vi "Keysight DAQ970-Example-Mantoles.vi"(5 "error in (no error)":errorcluster {"code" format="%.0x"}) -> (19 "error out":errorcluster)   [LabVIEW 2020, in "Keysight DAQ970.lvlib"]
doc: "Initializes the driver, reads a few Identity attributes, and checks the instrument error queue."
uses:
  Keysight DAQ970.lvlib
panel:
  out "Field Count":i32
  in  "MaxTimeMilliseconds":i32=5000
  in  "Sweep Count":i32=2 format="%.0g"
  in  "Resolution":dbl=0.01
  in  "Range":dbl=10.0
  out "muxSlot":i32=200
  out "dacSlot":i32=100
  out "Slot (Slot1)":i32
  out "Module ID":string
  out "ChannelList":string="(@305)"
  in  "Voltage":dbl=2.345
  out "Output":string
  out "Info":T1
  out "Simulate":bool
  in  "Simulate":bool=TRUE
  in  "Select ?":bool=TRUE
  in  "DAQ Resource":string="MyVisaAlias" caption="Instrument Resource"
  in  "Options String":string="DriverSetup= "
  # "Setup Scan"
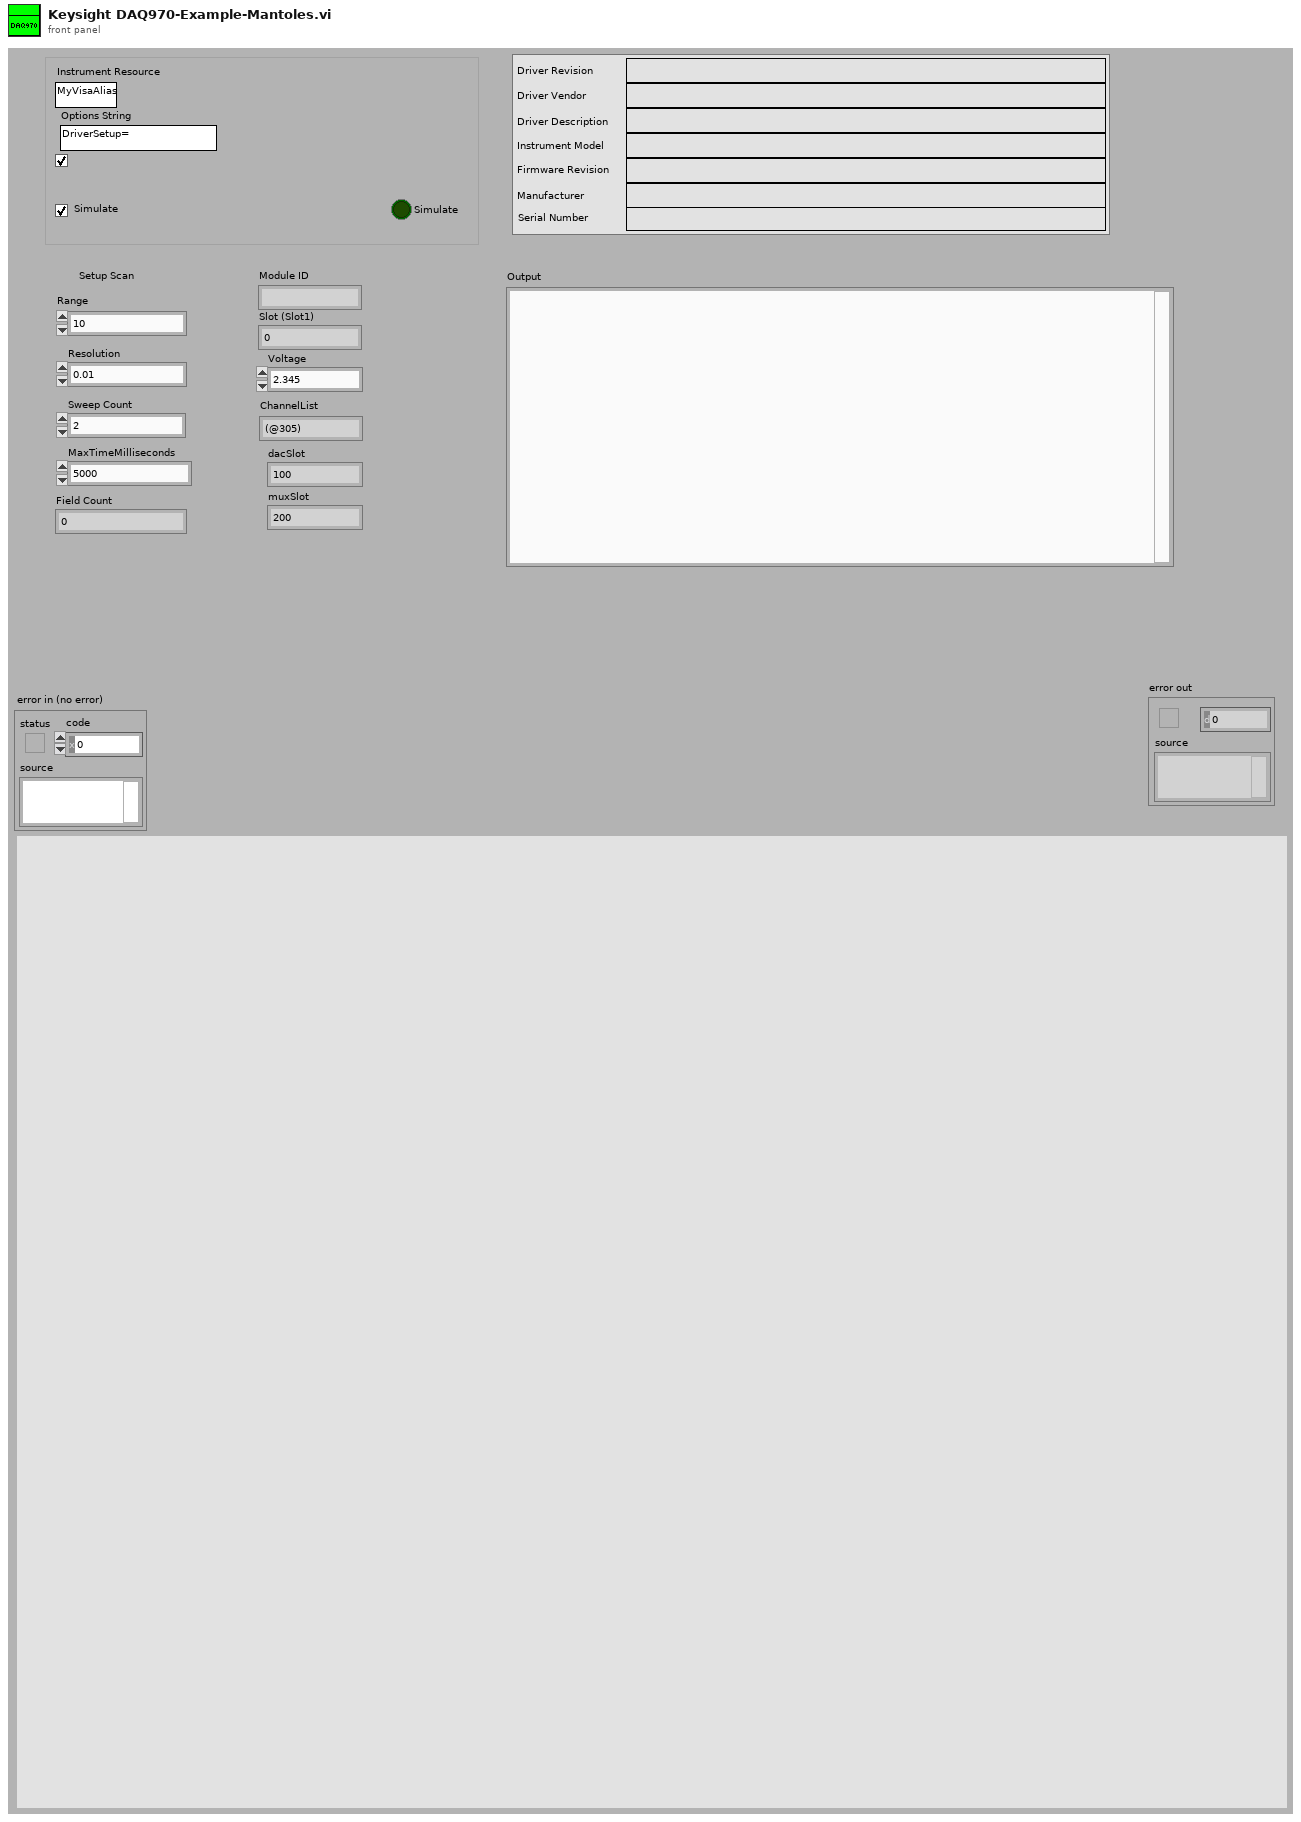
[diagram p1: front panel]
types:
  T1 = cluster{"Driver Revision":string, "Driver Vendor":string, "Driver Description":string, "Instrument Model":string, "Firmware Revision":string, "Instrument Model 2":string, "Firmware Revision 2":string}
  T2 = cluster{"[0]":string, "[1]":string, "[2]":string, "[3]":string, "[4]":string, "[5]":string, "[6]":string}
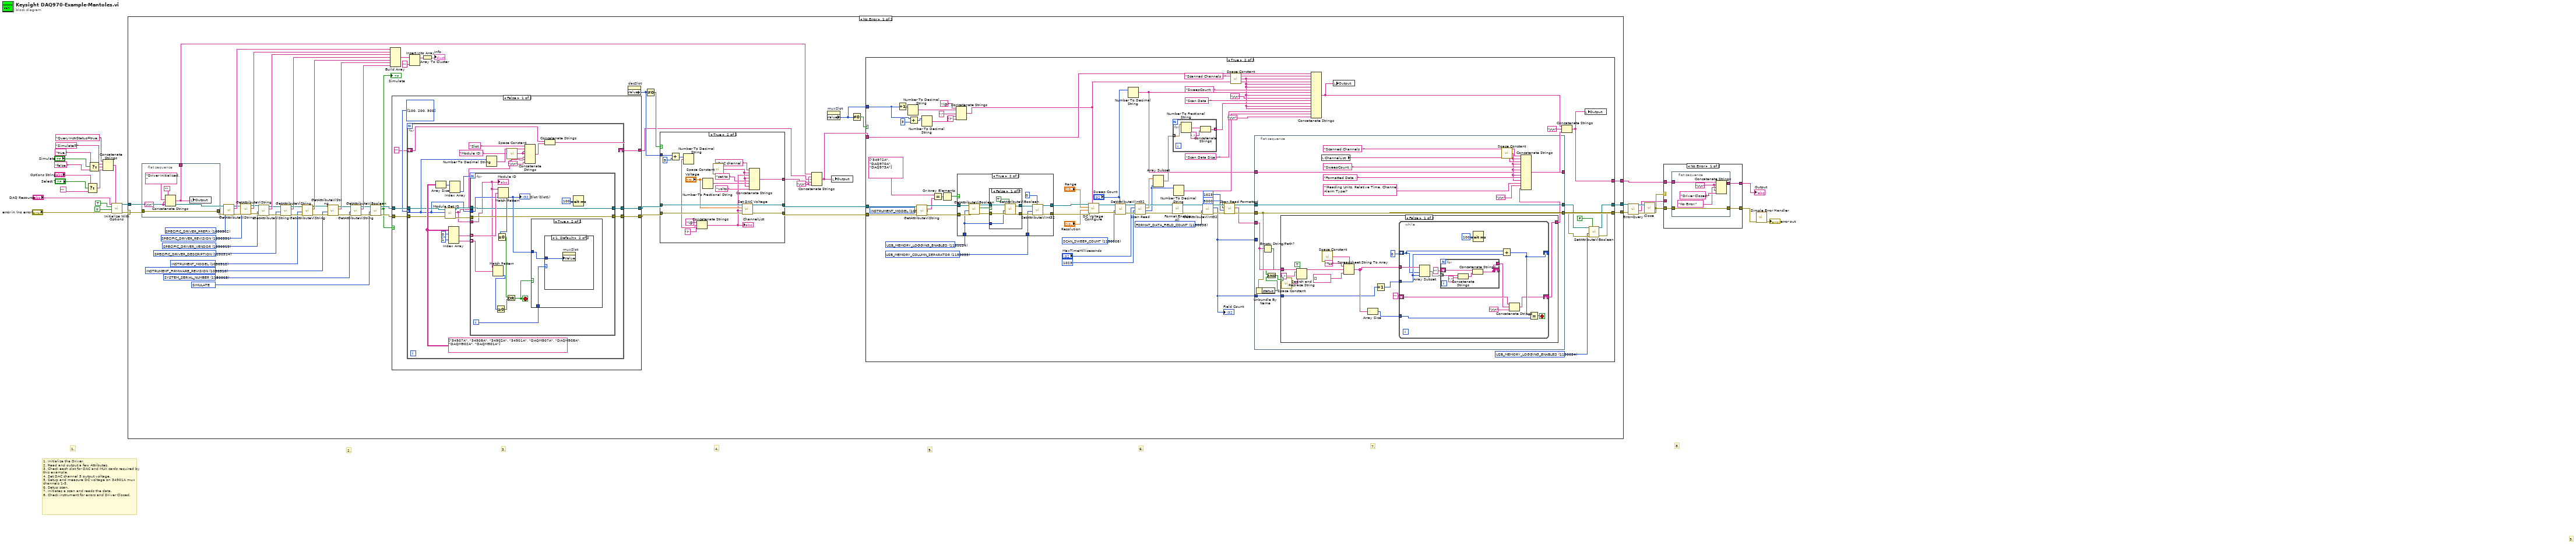
[diagram p0: block diagram]
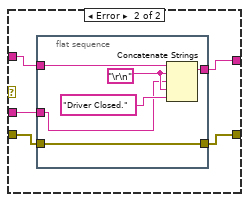
[diagram p2: hidden frame]
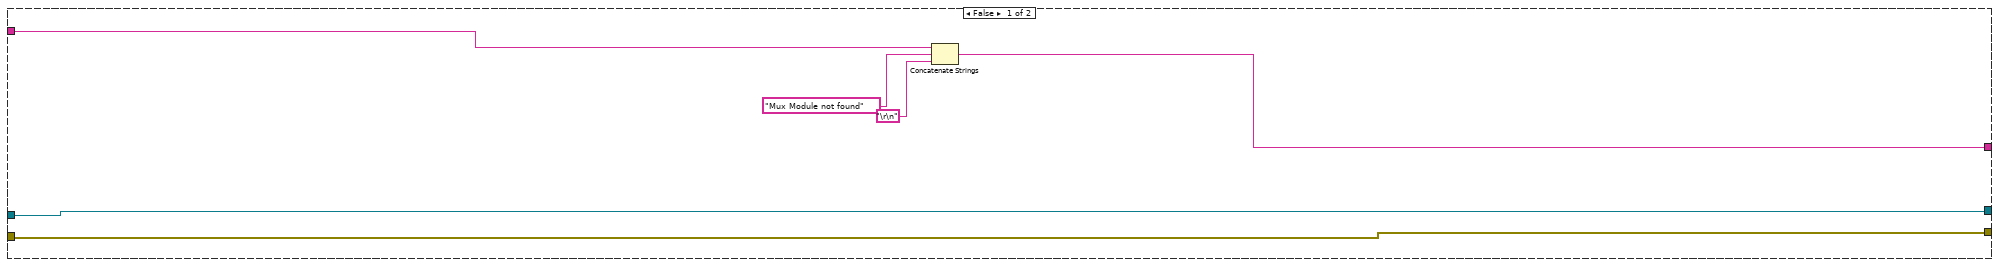
[diagram p3: hidden frame]
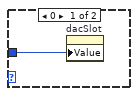
[diagram p8: hidden frame]
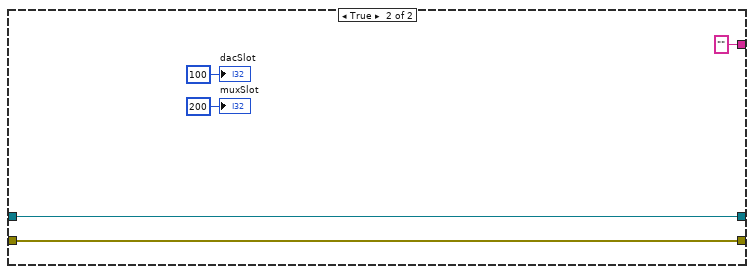
[diagram p9: hidden frame]
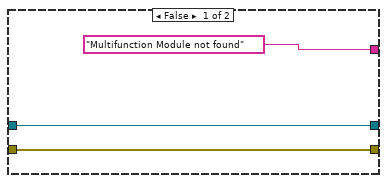
[diagram p10: hidden frame]
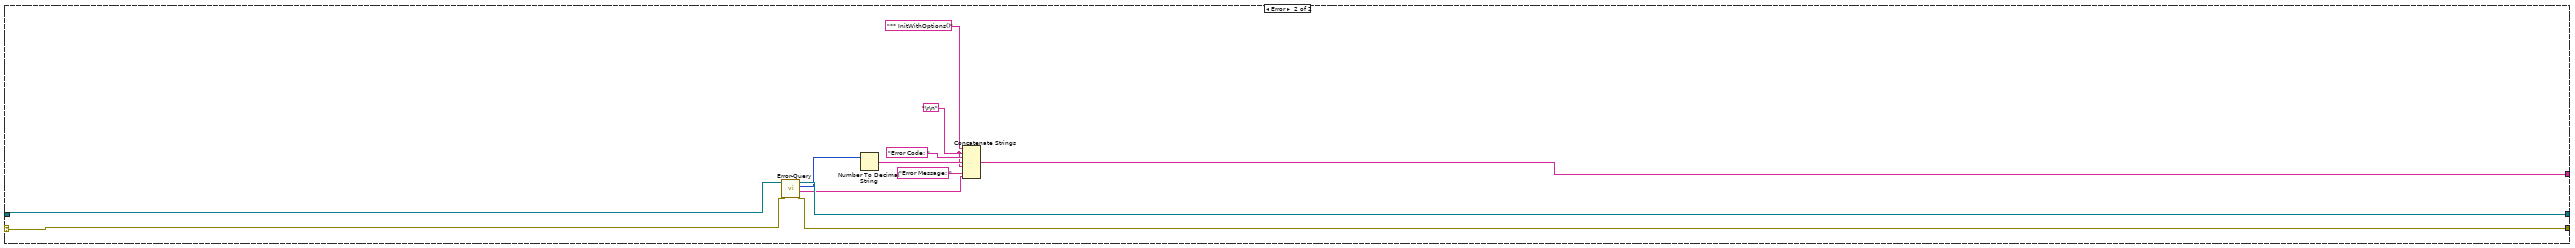
[diagram p11: hidden frame]
diagram:
  # "8."
  # "7."
  # "6."
  # "5."
  # "4."
  # "3."
  # "2."
  # "3."
  # "1."
  # "1. Initialize the Driver.\n2. Read and output a few Attributes.\n3. Check each slot for DAC and MUX cards required by this example.\n4. Set DAC channel 5 output voltage.\n5. Setup and measure DC voltage on 34901A mux channels 1-3.\n6. Setup scan. \n7. Initiates a scan and reads the data.\n8. Check instrument for errors and Driver Closed."
  n1 = Select(t="Options String", s="Select ?", f="") -> (s? t:f=w24:string)
  n2 = Select(t="true,", s="Simulate", f="false,") -> (s? t:f=w26:string)
  n3 = Concatenate Strings("QueryInstrStatus=true, " ("string"), "Simulate=" ("string"), w26, w24) -> (w16:string)
  n4 = call "Initialize With Options.vi"("option string"=w16, "error in (no error)"="error in (no error)", "reset device (Off)"=TRUE, "id query (Off)"=TRUE, "resource string"="DAQ Resource") -> ("error out"=w17:errorcluster, "instrument handle out"=w13:refnum<k15>)  [unwired: 5 in]
  n5 = case shown="No Error" w17 {
    selector: w17 -> [w82 w325]
    tunnel: [w33 w324] -> w8
    tunnel: w13 -> [w77 w323]
    tunnel: [w34 w322] -> w7
    tunnel: [w32 w314] -> w9
    frame No Error {
      w29 = "\r\n"
      w47 = u32 1050005 items=["DISPLAY_ENABLED"=1150016, "FORMAT_ALARM_ENABLED"=1150023, "FORMAT_CHANNEL_ENABLED"=1150024, "FORMAT_TIME_ENABLED"=1150025, "FORMAT_UNITS_ENABLED"=1150027, "ROUTE_MONITOR_ENABLED"=1150012, "SIMULATE"=1050005, "SYSTEM_AUTOCALIBRATION_GET_ALL_MODULE_STATE"=1150051, "SYSTEM_DMM_ENABLED"=1150018, "SYSTEM_DMM_INSTALLED"=1150019, "SYSTEM_INSTRUMENT_STATE_POWER_ON_RECALL_ENABLED"=1150033, "SYSTEM_LXI_IDENTIFY_ENABLED"=1150032, "SYSTEM_TRACING_ENABLED"=1150041, "USB_MEMORY_LOGGING_ENABLED"=1150034, "USB_MEMORY_MEASUREMENT_DATA_AUTO_SAVE_ENABLED"=1150057, "USB_MEMORY_RECALL_AUTO_ENABLED"=1150052, "USB_MEMORY_ROW_LIMIT_ENABLED"=1150036] ("AttributeID")
      w48 = u32 1150003 items=["CALIBRATION_DATE"=1150065, "CALIBRATION_MESSAGE"=1150015, "CALIBRATION_TIME"=1150066, "DISPLAY_TEXT"=1150017, "DRIVER_SETUP"=1050007, "GROUP_CAPABILITIES"=1050401, "INSTRUMENT_FIRMWARE_REVISION"=1050510, "INSTRUMENT_MANUFACTURER"=1050511, "INSTRUMENT_MODEL"=1050512, "IO_RESOURCE_DESCRIPTOR"=1050304, "LOGICAL_NAME"=1050305, "ROUTE_MONITOR_CHANNEL"=1150010, "SCAN_LIST"=1150004, "SCAN_STARTTIME"=1150022, "SPECIFIC_DRIVER_DESCRIPTION"=1050514, "SPECIFIC_DRIVER_PREFIX"=1050302, "SPECIFIC_DRIVER_REVISION"=1050551, "SPECIFIC_DRIVER_VENDOR"=1050513, "SUPPORTED_INSTRUMENT_MODELS"=1050327, "SYSTEM_DATE"=1150020, "SYSTEM_SERIAL_NUMBER"=1150003, "SYSTEM_TIME"=1150021, "SYSTEM_TRACING_FILE_NAME"=1150042, "USB_MEMORY_DATA_FILE"=1150056, "USB_MEMORY_MEASUREMENTS_DATA_AUTO_SAVE_FILE"=1150058, "USB_MEMORY_SELECT_RECALL_AUTO_FILE"=1150053] ("AttributeID")
      w49 = u32 1050510 items=["CALIBRATION_DATE"=1150065, "CALIBRATION_MESSAGE"=1150015, "CALIBRATION_TIME"=1150066, "DISPLAY_TEXT"=1150017, "DRIVER_SETUP"=1050007, "GROUP_CAPABILITIES"=1050401, "INSTRUMENT_FIRMWARE_REVISION"=1050510, "INSTRUMENT_MANUFACTURER"=1050511, "INSTRUMENT_MODEL"=1050512, "IO_RESOURCE_DESCRIPTOR"=1050304, "LOGICAL_NAME"=1050305, "ROUTE_MONITOR_CHANNEL"=1150010, "SCAN_LIST"=1150004, "SCAN_STARTTIME"=1150022, "SPECIFIC_DRIVER_DESCRIPTION"=1050514, "SPECIFIC_DRIVER_PREFIX"=1050302, "SPECIFIC_DRIVER_REVISION"=1050551, "SPECIFIC_DRIVER_VENDOR"=1050513, "SUPPORTED_INSTRUMENT_MODELS"=1050327, "SYSTEM_DATE"=1150020, "SYSTEM_SERIAL_NUMBER"=1150003, "SYSTEM_TIME"=1150021, "SYSTEM_TRACING_FILE_NAME"=1150042, "USB_MEMORY_DATA_FILE"=1150056, "USB_MEMORY_MEASUREMENTS_DATA_AUTO_SAVE_FILE"=1150058, "USB_MEMORY_SELECT_RECALL_AUTO_FILE"=1150053] ("AttributeID")
      w50 = u32 1050512 items=["CALIBRATION_DATE"=1150065, "CALIBRATION_MESSAGE"=1150015, "CALIBRATION_TIME"=1150066, "DISPLAY_TEXT"=1150017, "DRIVER_SETUP"=1050007, "GROUP_CAPABILITIES"=1050401, "INSTRUMENT_FIRMWARE_REVISION"=1050510, "INSTRUMENT_MANUFACTURER"=1050511, "INSTRUMENT_MODEL"=1050512, "IO_RESOURCE_DESCRIPTOR"=1050304, "LOGICAL_NAME"=1050305, "ROUTE_MONITOR_CHANNEL"=1150010, "SCAN_LIST"=1150004, "SCAN_STARTTIME"=1150022, "SPECIFIC_DRIVER_DESCRIPTION"=1050514, "SPECIFIC_DRIVER_PREFIX"=1050302, "SPECIFIC_DRIVER_REVISION"=1050551, "SPECIFIC_DRIVER_VENDOR"=1050513, "SUPPORTED_INSTRUMENT_MODELS"=1050327, "SYSTEM_DATE"=1150020, "SYSTEM_SERIAL_NUMBER"=1150003, "SYSTEM_TIME"=1150021, "SYSTEM_TRACING_FILE_NAME"=1150042, "USB_MEMORY_DATA_FILE"=1150056, "USB_MEMORY_MEASUREMENTS_DATA_AUTO_SAVE_FILE"=1150058, "USB_MEMORY_SELECT_RECALL_AUTO_FILE"=1150053] ("AttributeID")
      w51 = u32 1050514 items=["CALIBRATION_DATE"=1150065, "CALIBRATION_MESSAGE"=1150015, "CALIBRATION_TIME"=1150066, "DISPLAY_TEXT"=1150017, "DRIVER_SETUP"=1050007, "GROUP_CAPABILITIES"=1050401, "INSTRUMENT_FIRMWARE_REVISION"=1050510, "INSTRUMENT_MANUFACTURER"=1050511, "INSTRUMENT_MODEL"=1050512, "IO_RESOURCE_DESCRIPTOR"=1050304, "LOGICAL_NAME"=1050305, "ROUTE_MONITOR_CHANNEL"=1150010, "SCAN_LIST"=1150004, "SCAN_STARTTIME"=1150022, "SPECIFIC_DRIVER_DESCRIPTION"=1050514, "SPECIFIC_DRIVER_PREFIX"=1050302, "SPECIFIC_DRIVER_REVISION"=1050551, "SPECIFIC_DRIVER_VENDOR"=1050513, "SUPPORTED_INSTRUMENT_MODELS"=1050327, "SYSTEM_DATE"=1150020, "SYSTEM_SERIAL_NUMBER"=1150003, "SYSTEM_TIME"=1150021, "SYSTEM_TRACING_FILE_NAME"=1150042, "USB_MEMORY_DATA_FILE"=1150056, "USB_MEMORY_MEASUREMENTS_DATA_AUTO_SAVE_FILE"=1150058, "USB_MEMORY_SELECT_RECALL_AUTO_FILE"=1150053] ("AttributeID")
      w52 = u32 1050513 items=["CALIBRATION_DATE"=1150065, "CALIBRATION_MESSAGE"=1150015, "CALIBRATION_TIME"=1150066, "DISPLAY_TEXT"=1150017, "DRIVER_SETUP"=1050007, "GROUP_CAPABILITIES"=1050401, "INSTRUMENT_FIRMWARE_REVISION"=1050510, "INSTRUMENT_MANUFACTURER"=1050511, "INSTRUMENT_MODEL"=1050512, "IO_RESOURCE_DESCRIPTOR"=1050304, "LOGICAL_NAME"=1050305, "ROUTE_MONITOR_CHANNEL"=1150010, "SCAN_LIST"=1150004, "SCAN_STARTTIME"=1150022, "SPECIFIC_DRIVER_DESCRIPTION"=1050514, "SPECIFIC_DRIVER_PREFIX"=1050302, "SPECIFIC_DRIVER_REVISION"=1050551, "SPECIFIC_DRIVER_VENDOR"=1050513, "SUPPORTED_INSTRUMENT_MODELS"=1050327, "SYSTEM_DATE"=1150020, "SYSTEM_SERIAL_NUMBER"=1150003, "SYSTEM_TIME"=1150021, "SYSTEM_TRACING_FILE_NAME"=1150042, "USB_MEMORY_DATA_FILE"=1150056, "USB_MEMORY_MEASUREMENTS_DATA_AUTO_SAVE_FILE"=1150058, "USB_MEMORY_SELECT_RECALL_AUTO_FILE"=1150053] ("AttributeID")
      w53 = u32 1050551 items=["CALIBRATION_DATE"=1150065, "CALIBRATION_MESSAGE"=1150015, "CALIBRATION_TIME"=1150066, "DISPLAY_TEXT"=1150017, "DRIVER_SETUP"=1050007, "GROUP_CAPABILITIES"=1050401, "INSTRUMENT_FIRMWARE_REVISION"=1050510, "INSTRUMENT_MANUFACTURER"=1050511, "INSTRUMENT_MODEL"=1050512, "IO_RESOURCE_DESCRIPTOR"=1050304, "LOGICAL_NAME"=1050305, "ROUTE_MONITOR_CHANNEL"=1150010, "SCAN_LIST"=1150004, "SCAN_STARTTIME"=1150022, "SPECIFIC_DRIVER_DESCRIPTION"=1050514, "SPECIFIC_DRIVER_PREFIX"=1050302, "SPECIFIC_DRIVER_REVISION"=1050551, "SPECIFIC_DRIVER_VENDOR"=1050513, "SUPPORTED_INSTRUMENT_MODELS"=1050327, "SYSTEM_DATE"=1150020, "SYSTEM_SERIAL_NUMBER"=1150003, "SYSTEM_TIME"=1150021, "SYSTEM_TRACING_FILE_NAME"=1150042, "USB_MEMORY_DATA_FILE"=1150056, "USB_MEMORY_MEASUREMENTS_DATA_AUTO_SAVE_FILE"=1150058, "USB_MEMORY_SELECT_RECALL_AUTO_FILE"=1150053] ("AttributeID")
      w54 = u32 1050302 items=["CALIBRATION_DATE"=1150065, "CALIBRATION_MESSAGE"=1150015, "CALIBRATION_TIME"=1150066, "DISPLAY_TEXT"=1150017, "DRIVER_SETUP"=1050007, "GROUP_CAPABILITIES"=1050401, "INSTRUMENT_FIRMWARE_REVISION"=1050510, "INSTRUMENT_MANUFACTURER"=1050511, "INSTRUMENT_MODEL"=1050512, "IO_RESOURCE_DESCRIPTOR"=1050304, "LOGICAL_NAME"=1050305, "ROUTE_MONITOR_CHANNEL"=1150010, "SCAN_LIST"=1150004, "SCAN_STARTTIME"=1150022, "SPECIFIC_DRIVER_DESCRIPTION"=1050514, "SPECIFIC_DRIVER_PREFIX"=1050302, "SPECIFIC_DRIVER_REVISION"=1050551, "SPECIFIC_DRIVER_VENDOR"=1050513, "SUPPORTED_INSTRUMENT_MODELS"=1050327, "SYSTEM_DATE"=1150020, "SYSTEM_SERIAL_NUMBER"=1150003, "SYSTEM_TIME"=1150021, "SYSTEM_TRACING_FILE_NAME"=1150042, "USB_MEMORY_DATA_FILE"=1150056, "USB_MEMORY_MEASUREMENTS_DATA_AUTO_SAVE_FILE"=1150058, "USB_MEMORY_SELECT_RECALL_AUTO_FILE"=1150053] ("AttributeID")
      n6 = flat-sequence {
        tunnel: w82 -> [w313]
        tunnel: [w313] -> w76
        tunnel: [w309] -> w30
        frame #0 {
          w310 = "\r\n"
          n7 = Concatenate Strings("", "Driver Initialized.", w310, w310) -> (w309:string)
          n8 = local write "Output"(w309) -> ()
        }
      }
      n9 = call "GetAttributeViString.vi"("error in (no error)"=w76, "AttributeID"=w54, "instrument handle"=w77) -> ("error out"=w75:errorcluster, "AttributeValue"=w74:string, "instrument handle out"=w73:refnum<k15>)  [unwired: 6 in]
      n10 = call "GetAttributeViString.vi"("error in (no error)"=w75, "AttributeID"=w53, "instrument handle"=w73) -> ("error out"=w72:errorcluster, "AttributeValue"=w71:string, "instrument handle out"=w70:refnum<k15>)  [unwired: 6 in]
      n11 = call "GetAttributeViString.vi"("error in (no error)"=w72, "AttributeID"=w52, "instrument handle"=w70) -> ("error out"=w67:errorcluster, "AttributeValue"=w69:string, "instrument handle out"=w68:refnum<k15>)  [unwired: 6 in]
      n12 = call "GetAttributeViString.vi"("error in (no error)"=w67, "AttributeID"=w51, "instrument handle"=w68) -> ("error out"=w65:errorcluster, "AttributeValue"=w66:string, "instrument handle out"=w64:refnum<k15>)  [unwired: 6 in]
      n13 = call "GetAttributeViString.vi"("error in (no error)"=w65, "AttributeID"=w50, "instrument handle"=w64) -> ("error out"=w62:errorcluster, "AttributeValue"=w63:string, "instrument handle out"=w61:refnum<k15>)  [unwired: 6 in]
      n14 = call "GetAttributeViString.vi"("error in (no error)"=w62, "AttributeID"=w49, "instrument handle"=w61) -> ("error out"=w58:errorcluster, "AttributeValue"=w60:string, "instrument handle out"=w59:refnum<k15>)  [unwired: 6 in]
      n15 = call "GetAttributeViString.vi"("error in (no error)"=w58, "AttributeID"=w48, "instrument handle"=w59) -> ("error out"=w55:errorcluster, "AttributeValue"=w57:string, "instrument handle out"=w56:refnum<k15>)  [unwired: 6 in]
      n16 = call "GetAttributeViBoolean.vi"("error in (no error)"=w55, "AttributeID"=w47, "instrument handle"=w56) -> ("error out"=w45:errorcluster, "AttributeValue"=w44:bool, "instrument handle out"=w46:refnum<k15>)  [unwired: 6 in]
      "Simulate" <- w44
      n17 = Build Array(w74, w71, w69, w66, w63, w60, w57) -> (w79:string[])
      n18 = case shown="False" w44 {
        tunnel: w46 -> [w242 w287]
        tunnel: w45 -> [w241 w286]
        tunnel: [w240 w286] -> w40
        tunnel: [w239 w287] -> w41
        tunnel: [w237 "" ("string")] -> w28
        frame False {
          w238 = i32[] [100, 200, 300] items=["Slot1"=100, "Slot2"=200, "Slot3"=300]
          n19 = for {
            tunnel: w241 -> [w254]
            tunnel: w242 -> [w256]
            tunnel: w238 -> [w247] mode=indexing
            tunnel: [w265] -> w240
            tunnel: [w264] -> w239
            shift-right: [w243] -> w237
            shift-left: "" ("string") -> [w244]
            w261 = string[][] [["34907A", "34908A", "34902A", "34901A"], ["DAQM907A", "DAQM908A", "DAQM902A", "DAQM901A"]]
            n20 = Array Size(array=w261) -> (size(s)=w263:i32[])
            n21 = call "Module Get ID.vi"("error in (no error)"=w254, "Slot (Slot1)"=w247, "instrument handle"=w256) -> ("error out"=w253:errorcluster, "Val"=w245:string, "instrument handle out"=w255:refnum<k15>)  [unwired: 6 in]
            n22 = Index Array(array=w261, index (row) #1=0 ("index (row)"), index (row) #2=1 ("index (row)")) -> (element #1=w260:string[], element #2=w259:string[])  [unwired: 2 in]
            n23 = Index Array(array=w263) -> (element #2=w262:i32)  [unwired: 2 in, 1 out]
            n24 = for {
              N: w262 -> [_]
              tunnel: w247 -> [w269]
              tunnel: [w267] -> w265
              tunnel: [w268] -> w264
              tunnel: w260 -> [w275] mode=indexing
              tunnel: w259 -> [w273] mode=indexing
              tunnel: w255 -> [w268]
              tunnel: w253 -> [w267]
              tunnel: w245 -> [w266]
              i -> [w276]
              stop <- w270 stop-if-true
              n25 = Match Pattern(string=w266, regular expression=w273) -> (offset past match=w272:i32)  [unwired: 1 in, 3 out]
              n26 = Greater Or Equal To 0?(x=w272) -> (x >= 0?=w271:bool)
              n27 = Match Pattern(string=w266, regular expression=w275) -> (offset past match=w274:i32)  [unwired: 1 in, 3 out]
              n28 = Greater Or Equal To 0?(x=w274) -> (x >= 0?=w278:bool)
              n29 = Or(x=w278, y=w271) -> (x .or. y?=w270:bool)
              n30 = case shown="True" w270 {
                tunnel: w276 -> [_ w279]
                tunnel: w269 -> [_ w280]
                frame False {
                }
                frame True {
                  n31 = case shown="1, Default" w279 {
                    tunnel: w280 -> [w281 w282]
                    frame 0 {
                      n32 = property on="dacSlot" class="DigNum (strict)"("Value"=w281) -> ()  [unwired: 2 in, 2 out]
                    }
                    frame 1, Default {
                      n33 = property on="muxSlot" class="DigNum (strict)"("Value"=w282) -> ()  [unwired: 2 in, 2 out]
                    }
                  }
                }
              }
              n34 = Wait (ms)(milliseconds to wait=u32 100) -> ()  [unwired: 1 out]
              "Module ID" <- w266
              "Slot (Slot1)" <- w269
            }
            n35 = Number To Decimal String(number=w247) -> (decimal integer string=w251:string)  [unwired: 1 in]
            n36 = call <vilib>:"Space Constant.vi"() -> ("String"=w249:string)
            n37 = Concatenate Strings("Slot: " ("string"), w251, w249, w249, "Module ID: " ("string"), w245, "\r\n") -> (w252:string)
            n38 = Concatenate Strings(w244, w252) -> (w243:string)
          }
        }
        frame True {
          "dacSlot" <- 100 ("dacSlot")
          "muxSlot" <- 200 ("muxSlot")
        }
      }
      n39 = Insert Into Array(array=w79, new element="" ("new element/subarray")) -> (w80:string[])  [unwired: 1 in]
      n40 = Array To Cluster(array=w80) -> (cluster=→"Info":T2)
      n41 = property on="dacSlot" class="DigNum (strict)"() -> ("Value"=w42:i32)  [unwired: 2 in, 2 out]
      n42 = Not Equal To 0?(x=w42) -> (x != 0?=w43:bool)
      n43 = case shown="True" w43 {
        tunnel: w42 -> [_ w306]
        tunnel: w41 -> [w289 w305]
        tunnel: w40 -> [w288 w304]
        tunnel: ["Multifunction Module not found" ("new element/subarray") w300] -> w39
        tunnel: [w289 w299] -> w37
        tunnel: [w288 w298] -> w36
        frame False {
        }
        frame True {
          n44 = Add(x=w306, y=5 ("number")) -> (x+y=w307:i32)
          n45 = Number To Decimal String(number=w307) -> (decimal integer string=w296:string)  [unwired: 1 in]
          n46 = Concatenate Strings("(@" ("string"), w296, ")" ("string")) -> (w294:string)
          "ChannelList" <- w294
          n47 = Number To Fractional String(number="Voltage") -> (F-format string=w301:string)  [unwired: 3 in]
          n48 = call <vilib>:"Space Constant.vi"() -> ("String"=w291:string)
          n49 = call "Set DAC Voltage.vi"("error in (no error)"=w304, "ChannelList"=w294, "Voltage"="Voltage", "instrument handle"=w305) -> ("error out"=w298:errorcluster, "instrument handle out"=w299:refnum<k15>)  [unwired: 6 in]
          n50 = Concatenate Strings("DAC channel " ("new element/subarray"), w291, w294, w291, "set to " ("new element/subarray"), w301, w291, "volts." ("new element/subarray")) -> (w300:string)
        }
      }
      n51 = Concatenate Strings(w30, w29, w28, w39, w29) -> (w31:string)
      n52 = property on="muxSlot" class="DigNum (strict)"() -> ("Value"=w35:i32)  [unwired: 2 in, 2 out]
      n53 = local write "Output"(w31) -> ()
      n54 = Not Equal To 0?(x=w35) -> (x != 0?=w38:bool)
      n55 = case shown="True" w38 {
        tunnel: w37 -> [w88 w157]
        tunnel: w36 -> [w87 w156]
        tunnel: w35 -> [_ w143]
        tunnel: [w88 w97] -> w34
        tunnel: [w87 w96] -> w33
        tunnel: [w83 w107] -> w32
        tunnel: w31 -> [w86 w105]
        frame False {
          n56 = Concatenate Strings(w86, "Mux Module not found", "\r\n") -> (w83:string)
        }
        frame True {
          w94 = u32 1050512 items=["CALIBRATION_DATE"=1150065, "CALIBRATION_MESSAGE"=1150015, "CALIBRATION_TIME"=1150066, "DISPLAY_TEXT"=1150017, "DRIVER_SETUP"=1050007, "INSTRUMENT_MANUFACTURER"=1050511, "INSTRUMENT_MODEL"=1050512, "IO_RESOURCE_DESCRIPTOR"=1050304, "LOGICAL_NAME"=1050305, "ROUTE_MONITOR_CHANNEL"=1150010, "SCAN_LIST"=1150004, "SCAN_STARTTIME"=1150022, "SPECIFIC_DRIVER_DESCRIPTION"=1050514, "SPECIFIC_DRIVER_PREFIX"=1050302, "SPECIFIC_DRIVER_REVISION"=1050551, "SPECIFIC_DRIVER_VENDOR"=1050513, "SUPPORTED_INSTRUMENT_MODELS"=1050327, "SYSTEM_DATE"=1150020, "SYSTEM_SERIAL_NUMBER"=1150003, "SYSTEM_TIME"=1150021, "SYSTEM_TRACING_FILE_NAME"=1150042, "USB_MEMORY_DATA_FILE"=1150056, "USB_MEMORY_MEASUREMENTS_DATA_AUTO_SAVE_FILE"=1150058, "USB_MEMORY_SELECT_RECALL_AUTO_FILE"=1150053] ("AttributeID")
          w95 = u32 1150034 items=["DISPLAY_ENABLED"=1150016, "FORMAT_ALARM_ENABLED"=1150023, "FORMAT_CHANNEL_ENABLED"=1150024, "FORMAT_TIME_ENABLED"=1150025, "FORMAT_UNITS_ENABLED"=1150027, "ROUTE_MONITOR_ENABLED"=1150012, "SIMULATE"=1050005, "SYSTEM_DMM_ENABLED"=1150018, "SYSTEM_INSTRUMENT_STATE_POWER_ON_RECALL_ENABLED"=1150033, "SYSTEM_LXI_IDENTIFY_ENABLED"=1150032, "SYSTEM_TRACING_ENABLED"=1150041, "USB_MEMORY_LOGGING_ENABLED"=1150034, "USB_MEMORY_MEASUREMENT_DATA_AUTO_SAVE_ENABLED"=1150057, "USB_MEMORY_RECALL_AUTO_ENABLED"=1150052, "USB_MEMORY_ROW_LIMIT_ENABLED"=1150036] ("AttributeID")
          w127 = u32 1150038 items=["ALARM_MODE"=1150006, "ALARM_SLOPE"=1150007, "CALIBRATION_COUNT"=1150014, "FORMAT_DATA_FIELD_COUNT"=1150038, "FORMAT_TIME_MODE"=1150026, "ROUTE_MONITOR_VIEW"=1150068, "SCAN_CHANNEL_ADVANCE_SOURCE"=1150028, "SCAN_READING_COUNT"=1150030, "SCAN_READING_THRESHOLD"=1150031, "SCAN_SINGLE_CHANNEL_SAMPLE_COUNT_PRE_TRIGGER"=1150063, "SCAN_SINGLE_CHANNEL_SAMPLE_COUNT"=1150062, "SCAN_SIZE"=1150005, "SCAN_SWEEP_COUNT"=1150008, "SCAN_TRIGGER_OUTPUT_SLOPE"=1150067, "SCAN_TRIGGER_SLOPE"=1150061, "SCAN_TRIGGER_SOURCE"=1150009, "STATUS_ALARM_ENABLE_REGISTER"=1150040, "STATUS_OPERATION_ENABLE_REGISTER"=1150044, "STATUS_QUESTIONABLE_ENABLE_REGISTER"=1150045, "STATUS_SERVICE_REQUEST_ENABLE_REGISTER"=1150047, "STATUS_STANDARD_EVENT_ENABLE_REGISTER"=1150046, "SYSTEM_AUTOCALIBRATION_MONTHLY_INTERVAL_DAY"=1150049, "SYSTEM_AUTOCALIBRATION_OCCURENCE_INTERVAL"=1150048, "SYSTEM_AUTOCALIBRATION_WEEKLY_INTERVAL_DAY"=1150050, "SYSTEM_IO_TIMEOUT"=1150002, "SYSTEM_TRACING_LEVEL"=1150043, "USB_MEMORY_COLUMN_HEADER"=1150054, "USB_MEMORY_COLUMN_SEPARATOR"=1150035, "USB_MEMORY_ROW_LIMIT_COUNT"=1150055] ("AttributeID")
          w136 = u32 1150008 items=["ALARM_MODE"=1150006, "ALARM_SLOPE"=1150007, "FORMAT_TIME_MODE"=1150026, "ROUTE_MONITOR_VIEW"=1150068, "SCAN_CHANNEL_ADVANCE_SOURCE"=1150028, "SCAN_READING_THRESHOLD"=1150031, "SCAN_SINGLE_CHANNEL_SAMPLE_COUNT_PRE_TRIGGER"=1150063, "SCAN_SINGLE_CHANNEL_SAMPLE_COUNT"=1150062, "SCAN_SWEEP_COUNT"=1150008, "SCAN_TRIGGER_OUTPUT_SLOPE"=1150067, "SCAN_TRIGGER_SLOPE"=1150061, "SCAN_TRIGGER_SOURCE"=1150009, "STATUS_ALARM_ENABLE_REGISTER"=1150040, "STATUS_OPERATION_ENABLE_REGISTER"=1150044, "STATUS_QUESTIONABLE_ENABLE_REGISTER"=1150045, "STATUS_SERVICE_REQUEST_ENABLE_REGISTER"=1150047, "STATUS_STANDARD_EVENT_ENABLE_REGISTER"=1150046, "SYSTEM_AUTOCALIBRATION_MONTHLY_INTERVAL_DAY"=1150049, "SYSTEM_AUTOCALIBRATION_OCCURENCE_INTERVAL"=1150048, "SYSTEM_AUTOCALIBRATION_WEEKLY_INTERVAL_DAY"=1150050, "SYSTEM_IO_TIMEOUT"=1150002, "SYSTEM_TRACING_LEVEL"=1150043, "USB_MEMORY_COLUMN_HEADER"=1150054, "USB_MEMORY_COLUMN_SEPARATOR"=1150035, "USB_MEMORY_ROW_LIMIT_COUNT"=1150055] ("AttributeID")
          w152 = u32 1150035 items=["ALARM_MODE"=1150006, "ALARM_SLOPE"=1150007, "FORMAT_TIME_MODE"=1150026, "ROUTE_MONITOR_VIEW"=1150068, "SCAN_CHANNEL_ADVANCE_SOURCE"=1150028, "SCAN_READING_THRESHOLD"=1150031, "SCAN_SINGLE_CHANNEL_SAMPLE_COUNT_PRE_TRIGGER"=1150063, "SCAN_SINGLE_CHANNEL_SAMPLE_COUNT"=1150062, "SCAN_SWEEP_COUNT"=1150008, "SCAN_TRIGGER_OUTPUT_SLOPE"=1150067, "SCAN_TRIGGER_SLOPE"=1150061, "SCAN_TRIGGER_SOURCE"=1150009, "STATUS_ALARM_ENABLE_REGISTER"=1150040, "STATUS_OPERATION_ENABLE_REGISTER"=1150044, "STATUS_QUESTIONABLE_ENABLE_REGISTER"=1150045, "STATUS_SERVICE_REQUEST_ENABLE_REGISTER"=1150047, "STATUS_STANDARD_EVENT_ENABLE_REGISTER"=1150046, "SYSTEM_AUTOCALIBRATION_MONTHLY_INTERVAL_DAY"=1150049, "SYSTEM_AUTOCALIBRATION_OCCURENCE_INTERVAL"=1150048, "SYSTEM_AUTOCALIBRATION_WEEKLY_INTERVAL_DAY"=1150050, "SYSTEM_IO_TIMEOUT"=1150002, "SYSTEM_TRACING_LEVEL"=1150043, "USB_MEMORY_COLUMN_HEADER"=1150054, "USB_MEMORY_COLUMN_SEPARATOR"=1150035, "USB_MEMORY_ROW_LIMIT_COUNT"=1150055] ("AttributeID")
          w153 = u32 1150034 items=["DISPLAY_ENABLED"=1150016, "FORMAT_ALARM_ENABLED"=1150023, "FORMAT_CHANNEL_ENABLED"=1150024, "FORMAT_TIME_ENABLED"=1150025, "FORMAT_UNITS_ENABLED"=1150027, "ROUTE_MONITOR_ENABLED"=1150012, "SIMULATE"=1050005, "SYSTEM_AUTOCALIBRATION_GET_ALL_MODULE_STATE"=1150051, "SYSTEM_DMM_ENABLED"=1150018, "SYSTEM_DMM_INSTALLED"=1150019, "SYSTEM_INSTRUMENT_STATE_POWER_ON_RECALL_ENABLED"=1150033, "SYSTEM_LXI_IDENTIFY_ENABLED"=1150032, "SYSTEM_TRACING_ENABLED"=1150041, "USB_MEMORY_LOGGING_ENABLED"=1150034, "USB_MEMORY_MEASUREMENT_DATA_AUTO_SAVE_ENABLED"=1150057, "USB_MEMORY_RECALL_AUTO_ENABLED"=1150052, "USB_MEMORY_ROW_LIMIT_ENABLED"=1150036] ("AttributeID")
          n57 = Increment(x=w143) -> (x+1=w147:i32)
          n58 = Number To Decimal String(number=w147) -> (decimal integer string=w145:string)  [unwired: 1 in]
          n59 = Add(x=w143, y=3) -> (x+y=w141:i32)
          n60 = call "GetAttributeViString.vi"("error in (no error)"=w156, "AttributeID"=w94, "instrument handle"=w157) -> ("error out"=w154:errorcluster, "AttributeValue"=w93:string, "instrument handle out"=w155:refnum<k15>)  [unwired: 6 in]
          n61 = Number To Decimal String(number=w141) -> (decimal integer string=w140:string)  [unwired: 1 in]
          n62 = Equal?(x=string[] ["34972A", "DAQ970A", "DAQ973A"], y=w93) -> (x = y?=w92:bool[])
          n63 = Or Array Elements(Boolean array=w92) -> (logical OR=w91:bool)
          n64 = Concatenate Strings("(@" ("string"), w145, ":" ("string"), w140, ")" ("string")) -> (w102:string)
          n65 = case shown="True" w91 {
            tunnel: w155 -> [w160 w172]
            tunnel: w154 -> [w159 w171]
            tunnel: w153 -> [_ w168]
            tunnel: w152 -> [_ w165]
            tunnel: [w160 w163] -> w151
            tunnel: [w159 w162] -> w150
            frame False {
            }
            frame True {
              n66 = call "GetAttributeViBoolean.vi"("error in (no error)"=w171, "AttributeID"=w168, "instrument handle"=w172) -> ("error out"=w169:errorcluster, "AttributeValue"=w161:bool, "instrument handle out"=w170:refnum<k15>)  [unwired: 6 in]
              n67 = case shown="False" w161 {
                tunnel: w170 -> [w178 w180]
                tunnel: w169 -> [w177 w179]
                tunnel: w168 -> [w176 _]
                tunnel: [w175 w180] -> w167
                tunnel: [w174 w179] -> w166
                frame False {
                  n68 = call "SetAttributeViBoolean.vi"("AttributeValue (Off)"=TRUE, "error in (no error)"=w177, "AttributeID"=w176, "instrument handle"=w178) -> ("error out"=w174:errorcluster, "instrument handle out"=w175:refnum<k15>)  [unwired: 6 in]
                }
                frame True {
                }
              }
              n69 = call "SetAttributeViInt32.vi"("AttributeValue"=0, "error in (no error)"=w166, "AttributeID"=w165, "instrument handle"=w167) -> ("error out"=w162:errorcluster, "instrument handle out"=w163:refnum<k15>)  [unwired: 6 in]
            }
          }
          n70 = call "DC Voltage Configure.vi"("ChannelList"=w102, "error in (no error)"=w150, "Resolution"="Resolution", "Range"="Range", "instrument handle"=w151) -> ("error out"=w137:errorcluster, "instrument handle out"=w138:refnum<k15>)  [unwired: 5 in]
          n71 = call "SetAttributeViInt32.vi"("AttributeValue"="Sweep Count", "error in (no error)"=w137, "AttributeID"=w136, "instrument handle"=w138) -> ("error out"=w134:errorcluster, "instrument handle out"=w135:refnum<k15>)  [unwired: 6 in]
          n72 = Number To Decimal String(number="Sweep Count") -> (decimal integer string=w104:string)  [unwired: 1 in]
          n73 = call "Scan Read.vi"("error in (no error)"=w134, "ValBufferSize"=1023, "MaxTimeMilliseconds"="MaxTimeMilliseconds", "instrument handle"=w135) -> ("error out"=w130:errorcluster, "ValActualSize"=w116:i32, "Val"=w132:dbl[], "instrument handle out"=w131:refnum<k15>)  [unwired: 4 in]
          n74 = Array Subset(array=w132, length=w116) -> (w121:dbl[])  [unwired: 1 in]
          n75 = call "Format Enable All.vi"("error in (no error)"=w130, "instrument handle"=w131) -> ("error out"=w128:errorcluster, "instrument handle out"=w129:refnum<k15>)  [unwired: 8 in]
          n76 = for {
            tunnel: w121 -> [w235] mode=indexing
            tunnel: [w232] -> w120 mode=indexing
            n77 = Number To Fractional String(number=w235) -> (F-format string=w234:string)  [unwired: 3 in]
            n78 = Concatenate Strings(w234, "," ("string")) -> (w232:string)
          }
          n79 = Number To Decimal String(number=w116) -> (decimal integer string=w115:string)  [unwired: 1 in]
          n80 = call "GetAttributeViInt32.vi"("error in (no error)"=w128, "AttributeID"=w127, "instrument handle"=w129) -> ("error out"=w125:errorcluster, "AttributeValue"=w101:i32, "instrument handle out"=w126:refnum<k15>)  [unwired: 6 in]
          "Field Count" <- w101
          n81 = call "Scan Read Formatted.vi"("error in (no error)"=w125, "ValBufferSize"=1023, "MaxTimeMilliseconds"=5000, "instrument handle"=w126) -> ("error out"=w109:errorcluster, "Val"=w108:string, "instrument handle out"=w110:refnum<k15>)  [unwired: 5 in]
          n82 = call <vilib>:"Space Constant.vi"() -> ("String"=w118:string)
          n83 = flat-sequence {
            tunnel: [w197] -> w99
            tunnel: w110 -> [w197]
            tunnel: [w184] -> w98
            tunnel: w109 -> [w184]
            tunnel: w108 -> [w185]
            tunnel: w104 -> [w195]
            tunnel: [w191] -> w103
            tunnel: w101 -> [_]
            tunnel: w101 -> [w187]
            frame #0 {
              n84 = Unbundle By Name(w184) -> ("status"=w181:bool)
              n85 = Empty String/Path?(string/path=w185) -> (empty?=w182:bool)
              n86 = And(x=w182, y=w181) -> (x .and. y?=w183:bool)
              n87 = case shown="False" w183 {
                tunnel: w185 -> [w201 w231]
                tunnel: w187 -> [w200 _]
                tunnel: [w198 w231] -> w186
                frame False {
                  n88 = call <vilib>:"Space Constant.vi"() -> ("String"=w204:string)
                  n89 = Search and Replace String(replace all?=TRUE ("replace all? (F)"), input string=w201, search string=",", replace string=w204) -> (result string=w205:string)  [unwired: 4 in, 3 out]
                  n90 = call <vilib>:"Space Constant.vi"() -> ("String"=w208:string)
                  n91 = Spreadsheet String To Array(delimiter (Tab)=w208, format string="%s", spreadsheet string=w205, array type (2D Dbl)=string[] []) -> (array=w210:string[])
                  n92 = Array Size(array=w210) -> (size(s)=w211:i32)
                  n93 = Increment(x=w200) -> (x+1=w199:i32)
                  n94 = while {
                    tunnel: w210 -> [w225]
                    shift-right: [w220] -> _
                    shift-left: 0 ("index") -> [w213]
                    tunnel: w199 -> [w222]
                    tunnel: w211 -> [w219]
                    shift-right: [w216] -> w198
                    shift-left: "" ("string") -> [w217]
                    stop <- w218 stop-if-true
                    n95 = Array Subset(array=w225, index=w213, length=w222) -> (w223:string[])
                    n96 = for {
                      tunnel: w223 -> [w230] mode=indexing
                      shift-right: [w226] -> _
                      shift-left: "" ("string") -> [w228]
                      tunnel: [w226] -> w214
                      n97 = Concatenate Strings(w230, "," ("string")) -> (w227:string)
                      n98 = Concatenate Strings(w228, w227) -> (w226:string)
                    }
                    n99 = Wait (ms)(milliseconds to wait=u32 100) -> ()  [unwired: 1 out]
                    n100 = Add(x=w213, y=w222) -> (x+y=w220:i32)
                    n101 = Concatenate Strings(w217, w214, "\r\n") -> (w216:string)
                    n102 = Equal?(x=w220, y=w219) -> (x = y?=w218:bool)
                  }
                }
                frame True {
                }
              }
              n103 = local read "ChannelList"() -> (w190:string)
              n104 = call <vilib>:"Space Constant.vi"() -> ("String"=w188:string)
              n105 = Concatenate Strings("Scanned Channels : " ("string"), w188, w190, w188, "SweepCount : " ("string"), w188, w195, w188, "Formatted Data : " ("string"), w188, "(Reading Units, Relative Time, Channel, Alarm Type)" ("string"), "\r\n", w186) -> (w191:string)
            }
          }
          n106 = Concatenate Strings(w105, "Scanned Channels : " ("string"), w118, w102, w118, w118, "SweepCount : " ("string"), w104, w118, "\r\n", "Scan Data : " ("string"), w120, w118, w118, "Scan Data Size : " ("string"), w115, "\r\n") -> (w106:string)
          n107 = local write "Output"(w106) -> ()
          n108 = Concatenate Strings(w106, "\r\n", w103) -> (w107:string)
          n109 = local write "Output"(w107) -> ()
          n110 = call "SetAttributeViBoolean.vi"("AttributeValue (Off)"=FALSE, "error in (no error)"=w98, "AttributeID"=w95, "instrument handle"=w99) -> ("error out"=w96:errorcluster, "instrument handle out"=w97:refnum<k15>)  [unwired: 6 in]
        }
      }
    }
    frame Error {
      w315 = "\r\n"
      n111 = call "Error-Query.vi"("error in (no error)"=w325, "instrument handle"=w323) -> ("error out"=w324:errorcluster, "error message"=w321:string, "error code"=w319:i32, "instrument handle out"=w322:refnum<k15>)  [unwired: 6 in]
      n112 = Number To Decimal String(number=w319) -> (decimal integer string=w318:string)  [unwired: 1 in]
      n113 = Concatenate Strings("** InitWithOptions()" ("string"), w315, "Error Code: " ("string"), w318, w315, "Error Message: " ("string"), w321) -> (w314:string)
    }
  }
  n114 = call "Error-Query.vi"("error in (no error)"=w8, "instrument handle"=w7) -> ("error out"=w5:errorcluster, "error message"=w4:string, "instrument handle out"=w6:refnum<k15>)  [unwired: 6 in, 1 out]
  n115 = call "Close.vi"("error in (no error)"=w5, "instrument handle"=w6) -> ("error out"=w10:errorcluster)  [unwired: 9 in]
  n116 = case shown="No Error" w10 {
    tunnel: w10 -> [w329 w337]
    tunnel: [w328 w338] -> w12
    tunnel: [w327 w339] -> w11
    tunnel: w9 -> [w326 w340]
    tunnel: w4 -> [_ w336]
    frame No Error {
      n117 = flat-sequence {
        tunnel: w329 -> [w335]
        tunnel: [w335] -> w328
        tunnel: [w334] -> w327
        tunnel: w326 -> [w333]
        frame #0 {
          w330 = "\r\n"
          n118 = Concatenate Strings(w333, w330, "No Error.", w330, "Driver Closed.") -> (w334:string)
        }
      }
    }
    frame Error {
      n119 = flat-sequence {
        tunnel: w337 -> [w346]
        tunnel: [w346] -> w338
        tunnel: [w345] -> w339
        tunnel: w340 -> [w344]
        tunnel: w336 -> [w341]
        frame #0 {
          w342 = "\r\n"
          n120 = Concatenate Strings(w344, w342, w341, w342, "Driver Closed.") -> (w345:string)
        }
      }
    }
  }
  "Output" <- w11
  n121 = call <vilib>:"Simple Error Handler.vi"("error in (no error)"=w12) -> ("error out"=→"error out":errorcluster)  [unwired: 4 in, 4 out]
